vi "Pre-Build Custom Action.vi"(10 "Variant":variant) -> (0 "error out":errorcluster)   [LabVIEW 2013]
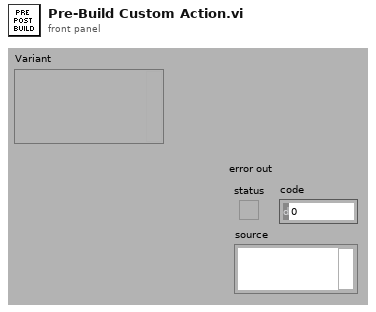
[diagram p1: front panel]
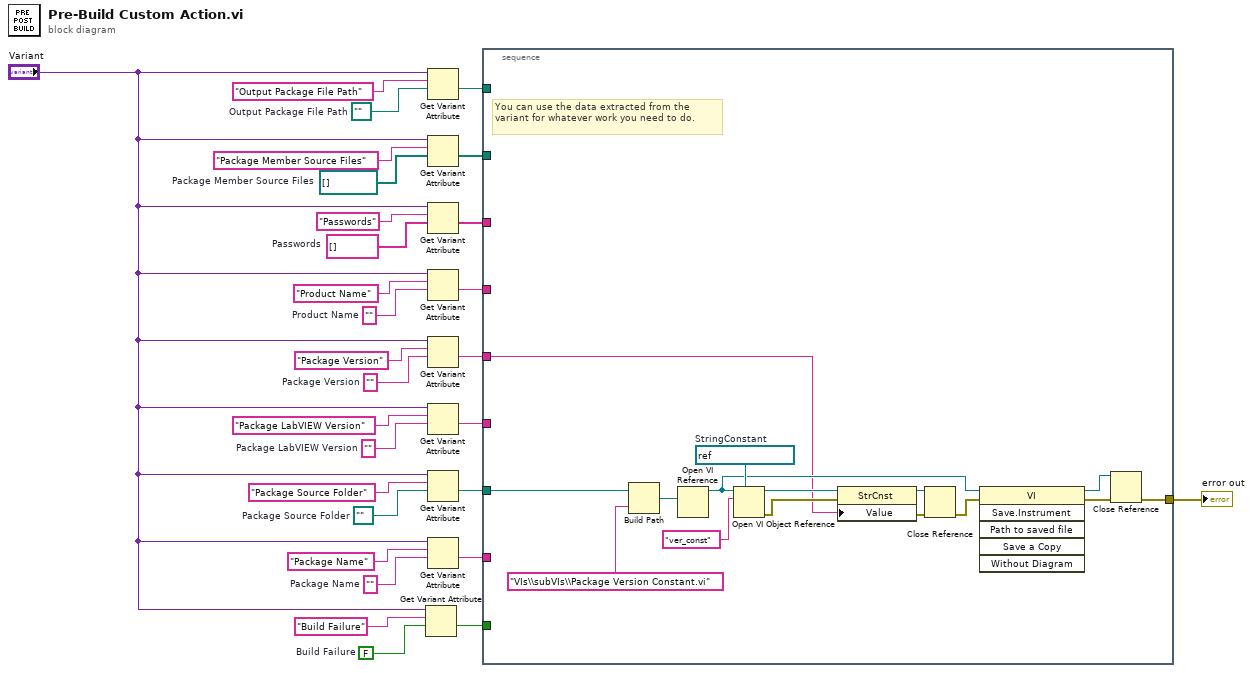
[diagram p0: block diagram]
diagram:
  w4 = FALSE  # Build Failure
  w14 = path ""  # Package Source Folder
  w15 = ""  # Package Name
  w18 = ""  # Package LabVIEW Version
  w20 = ""  # Package Version
  w22 = ""  # Product Name
  w24 = string[] []  # Passwords
  w26 = path[] []  # Package Member Source Files
  w28 = path ""  # Output Package File Path
  n1 = Get Variant Attribute(Variant="Variant", name="Build Failure", default value (empty Variant)=w4) -> (value=w2:bool)  [unwired: 1 in, 3 out]
  n2 = Get Variant Attribute(Variant="Variant", name="Output Package File Path", default value (empty Variant)=w28) -> (value=w13:path)  [unwired: 1 in, 3 out]
  n3 = Get Variant Attribute(Variant="Variant", name="Package Member Source Files", default value (empty Variant)=w26) -> (value=w12:path[])  [unwired: 1 in, 3 out]
  n4 = Get Variant Attribute(Variant="Variant", name="Passwords", default value (empty Variant)=w24) -> (value=w11:string[])  [unwired: 1 in, 3 out]
  n5 = Get Variant Attribute(Variant="Variant", name="Product Name", default value (empty Variant)=w22) -> (value=w10:string)  [unwired: 1 in, 3 out]
  n6 = Get Variant Attribute(Variant="Variant", name="Package Version", default value (empty Variant)=w20) -> (value=w9:string)  [unwired: 1 in, 3 out]
  n7 = Get Variant Attribute(Variant="Variant", name="Package LabVIEW Version", default value (empty Variant)=w18) -> (value=w8:string)  [unwired: 1 in, 3 out]
  n8 = Get Variant Attribute(Variant="Variant", name="Package Source Folder", default value (empty Variant)=w14) -> (value=w7:path)  [unwired: 1 in, 3 out]
  n9 = Get Variant Attribute(Variant="Variant", name="Package Name", default value (empty Variant)=w15) -> (value=w6:string)  [unwired: 1 in, 3 out]
  n10 = stacked-sequence {
    tunnel: w13 -> [_]
    tunnel: w12 -> [_]
    tunnel: w11 -> [_]
    tunnel: w10 -> [_]
    tunnel: w9 -> [w30]
    tunnel: w8 -> [_]
    tunnel: w7 -> [w35]
    tunnel: w6 -> [_]
    tunnel: w2 -> [_]
    tunnel: [w36] -> w1
    frame #0 {
      w44 = refnum<vi> refnum  # StringConstant
      # "You can use the data extracted from the variant for whatever work you need to do."
      n11 = Build Path(base path=w35, name or relative path="VIs\\subVIs\\Package Version Constant.vi") -> (appended path=w34:path)
      n12 = Open VI Reference(vi path=w34) -> (vi reference=w40:refnum<vi>)  [unwired: 5 in, 1 out]
      n13 = Open VI Object Reference(7:w44, 10:"ver_const" ("name/order"), 11:w40) -> (0:w37:errorcluster, 3:w41:refnum<vi>)  [unwired: 1 in]
      n14 = property class="StrCnst"(reference=w41, error in=w37, "Value"=w30) -> (reference out=w31:refnum<vi>, error out=w33:errorcluster)
      n15 = Close Reference(reference=w31, error in (no error)=w33) -> (error out=w32:errorcluster)
      n16 = invoke class="VI" method="Save.Instrument"(reference=w40, error in=w32) -> (reference out=w39:refnum<vi>, error out=w38:errorcluster)  [unwired: 4 in, 4 out]
      n17 = Close Reference(reference=w39, error in (no error)=w38) -> (error out=w36:errorcluster)
    }
  }
  "error out" <- w1
